vi "tb_magnitude_power_host.vi"() -> ()   [LabVIEW 2011]
uses:
  <vilib>/Analysis/NI_AALBase.lvlib
  <vilib>/measure/NI_MAPro.lvlib
  <vilib>/measure/maspectr.llb/FFT Spectrum (Mag-Phase) for 1 Chan.vi
panel:
  out "FPGA Output":dbl[](graph)
  out "Error Spectrum":cluster{"f0":dbl, "df":dbl, "magnitude":dbl[]}(graph)
  out "Error Signal":dbl[](graph)
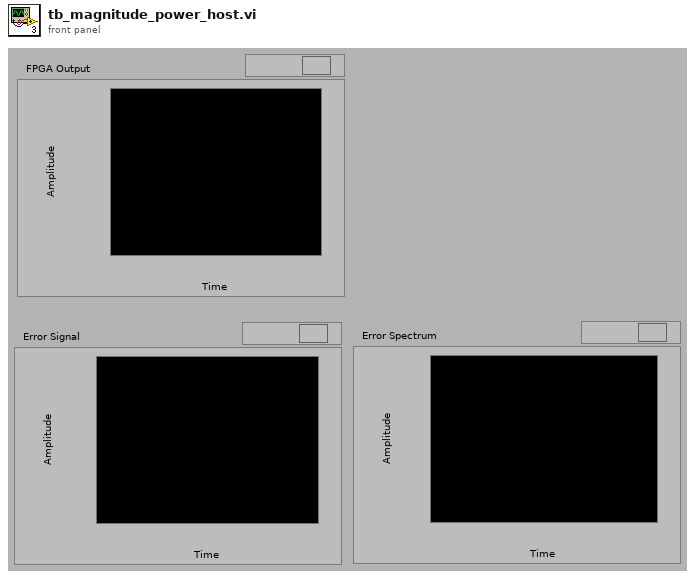
[diagram p1: front panel]
types:
  T1 = cluster{"dB On (F)":bool, "unwrap phase (F)":bool, "convert to degree (F)":bool}
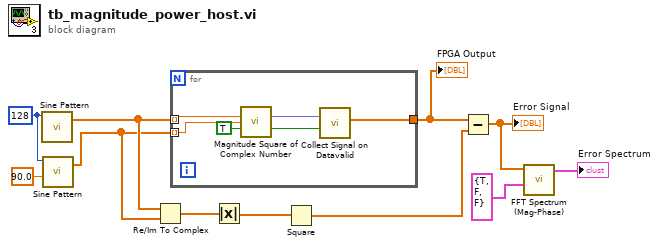
[diagram p0: block diagram]
diagram:
  w10 = 128 ("samples")
  n1 = call <vilib>:"Sine Pattern.vi"("samples"=w10) -> ("Sinusoidal Pattern"=w8:dbl[])  [unwired: 3 in, 1 out]
  n2 = call <vilib>:"Sine Pattern.vi"("phase(degrees)"=90.0, "samples"=w10) -> ("Sinusoidal Pattern"=w7:dbl[])  [unwired: 2 in, 1 out]
  n3 = Re/Im To Complex(1:w7, 2:w8) -> (0:w6:cdb[])
  n4 = for {
    tunnel: w8 -> [w16] mode=indexing
    tunnel: w7 -> [w15] mode=indexing
    tunnel: [w17] -> w1
    n5 = call "Magnitude Square of Complex Number.vi"("Real"=w16, "Imaginary"=w15, "Input Valid"=TRUE) -> ("Magnitude^2"=w12:fxp<+,48,14>, "Output Valid"=w13:bool)  [unwired: 11 in]
    n6 = call <userlib>:"Collect Signal on Datavalid.vi"("Data Valid"=w13, "Input"=w12) -> ("Output"=w17:dbl[])  [unwired: 9 in]
  }
  "FPGA Output" <- w1
  n7 = Absolute Value(x=w6) -> (abs(x)=w11:dbl[])
  n8 = Square(x=w11) -> (x^2=w5:dbl[])
  n9 = Subtract(x=w1, y=w5) -> (x-y=w4:dbl[])
  "Error Signal" <- w4
  n10 = call-poly <vilib>:"FFT Spectrum (Mag-Phase).vi"("view"=T1 {"dB On (F)"=TRUE, "unwrap phase (F)"=FALSE, "convert to degree (F)"=FALSE}, "time signal"=w4) -> ("magnitude"=→"Error Spectrum":cluster{"f0":dbl, "df":dbl, "magnitude":dbl[]})  [unwired: 5 in, 4 out]
